vi "Get latest folder based on date mod.vi"(11 "path":path) -> (3 "appended path":path)   [LabVIEW 2012]
panel:
  out "max index(es)":i32
  out "max value":timestamp
  out "folder names":string[](array[string])
  out "Array":timestamp[](array[timestamp])
  out "directory":bool
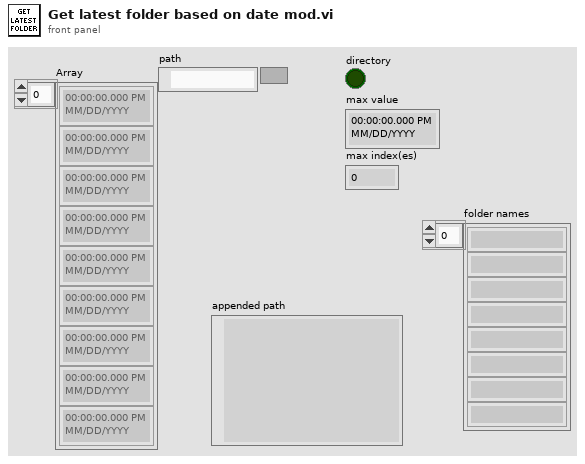
[diagram p1: front panel]
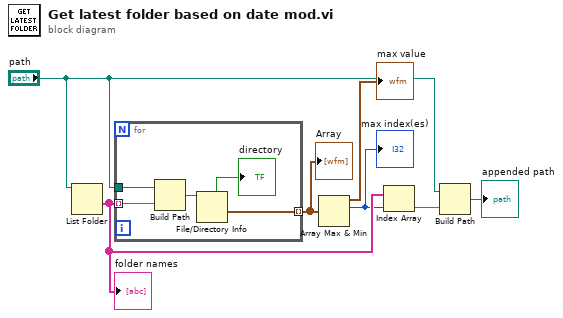
[diagram p0: block diagram]
diagram:
  n1 = List Folder(path="path") -> (folder names=w5:string[])  [unwired: 3 in, 3 out]
  "folder names" <- w5
  n2 = for {
    tunnel: "path" -> [w10]
    tunnel: [w11] -> w7 mode=indexing
    tunnel: w5 -> [w9] mode=indexing
    n3 = Build Path(base path=w10, name or relative path=w9) -> (appended path=w8:path)
    n4 = File/Directory Info(path=w8) -> (directory=→"directory":bool, last mod=w11:timestamp)  [unwired: 1 in, 5 out]
  }
  "Array" <- w7
  n5 = Array Max & Min(array=w7) -> (max value=→"max value":timestamp, max index (indices)=w4:i32)  [unwired: 2 out]
  "max index(es)" <- w4
  n6 = Index Array(array=w5, index=w4) -> (element=w3:string)
  n7 = Build Path(base path="path", name or relative path=w3) -> (appended path=→"appended path":path)
